vi "PBLV_Interface.vi"() -> ()   [LabVIEW 2012]
uses:
  <vilib>/Utility/error.llb/DialogTypeEnum.ctl
panel:
  in  "board_num":i32
  in  "change board":bool
  in  "# of Instructions":u32=4
  in  "Path to spinapi64.dll":path=path "C:/SpinCore/SpinAPI/dll/spinapi64.dll"
  in  "start/restart":bool
  in  "load":bool
  in  "stop":bool
  in  "clock_freq (MHz)":dbl=100.0
  in  "Instructions":T1(array[cluster])=[{"Instruct Data"=0, "Op Code"=0, "Flags"=[TRUE, FALSE, FALSE, FALSE, FALSE, FALSE, FALSE, FALSE, FALSE, FALSE, FALSE, FALSE, FALSE, FALSE, FALSE, FALSE, FALSE, FALSE, FALSE, FALSE, FALSE, FALSE, FALSE, FALSE], "Comments"="", "Time (s)"=0.1}, {"Instruct Data"=0, "Op Code"=0, "Flags"=[FALSE, FALSE, FALSE, FALSE, FALSE, FALSE, FALSE, FALSE, FALSE, FALSE, FALSE, FALSE, FALSE, FALSE, FALSE, FALSE, FALSE, FALSE, FALSE, FALSE, FALSE, FALSE, FALSE, FALSE], "Comments"="", "Time (s)"=0.1}, {"Instruct Data"=0, "Op Code"=0, "Flags"=[TRUE, FALSE, FALSE, FALSE, FALSE, FALSE, FALSE, FALSE, FALSE, FALSE, FALSE, FALSE, FALSE, FALSE, FALSE, FALSE, FALSE, FALSE, FALSE, FALSE, FALSE, FALSE, FALSE, FALSE], "Comments"="", "Time (s)"=0.1}, {"Instruct Data"=0, "Op Code"=6, "Flags"=[FALSE, FALSE, FALSE, FALSE, FALSE, FALSE, FALSE, FALSE, FALSE, FALSE, FALSE, FALSE, FALSE, FALSE, FALSE, FALSE, FALSE, FALSE, FALSE, FALSE, FALSE, FALSE, FALSE, FALSE], "Comments"="", "Time (s)"=0.1}] {"Time (s)" format="%.3p"; "Op Code" items=["Continue", "Stop", "Loop", "End Loop", "JSR", "RTS", "Branch", "Long Delay", "Wait"]}
  # "LabVIEW PulseBlaster Extension\nPulseBlaster Interface\nSpinCore Technologies, Inc.\nwww.spincore.com"
  # "Caution:    \n            After pressing STOP,\n            all output bits may \nmaintain their final state."
  # "1"
  # "2"
  # "3"
  # "4"
  # "5"
  # "6"
  # "7"
  # "8"
  # "9"
  # "10"
  # "11"
  # "12"
  # "13"
  # "14"
  # "15"
  # "16"
  # "17"
  # "18"
  # "19"
  # "20"
  # "21"
  # "22"
  # "23"
  # "24"
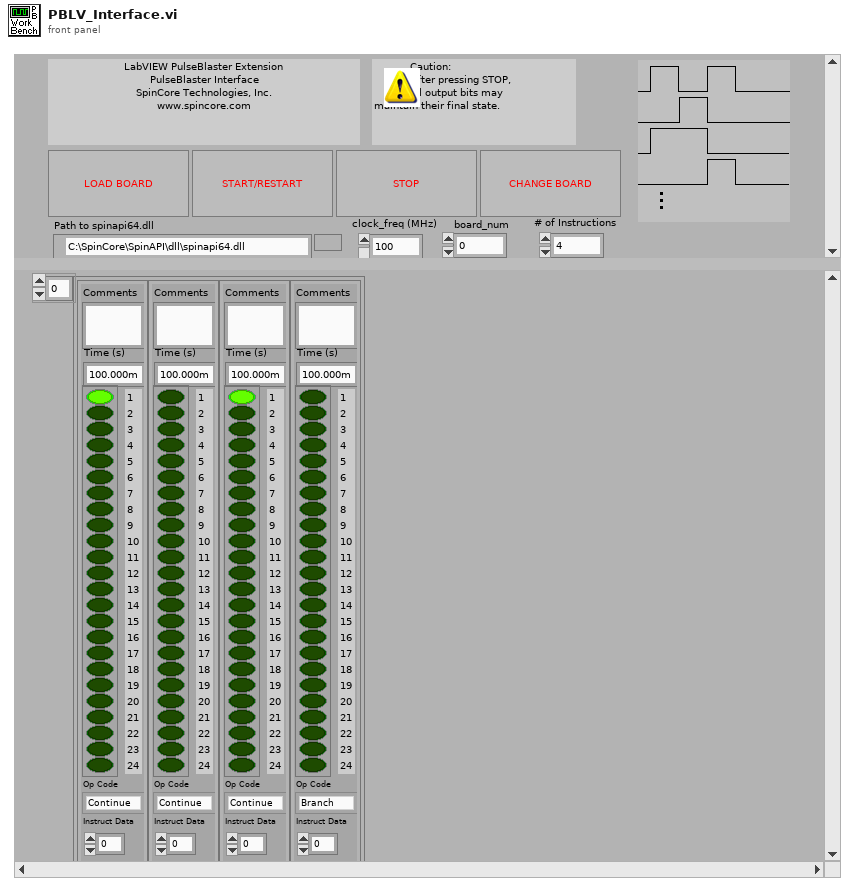
[diagram p1: front panel]
types:
  T1 = cluster{"Instruct Data":i32, "Op Code":i32, "Flags":bool[], "Comments":string, "Time (s)":dbl}[]
  T2 = typedef "DialogTypeEnum.ctl" = enum16{"no dialog", "OK message", "continue or stop message", "auto error handling dialog", "OK message + warnings", "continue/stop + warnings"}
  T3 = enum16{"Pulse Program", "Frequency Registers", "TX Phase Registers", "RX Phase Registers"}
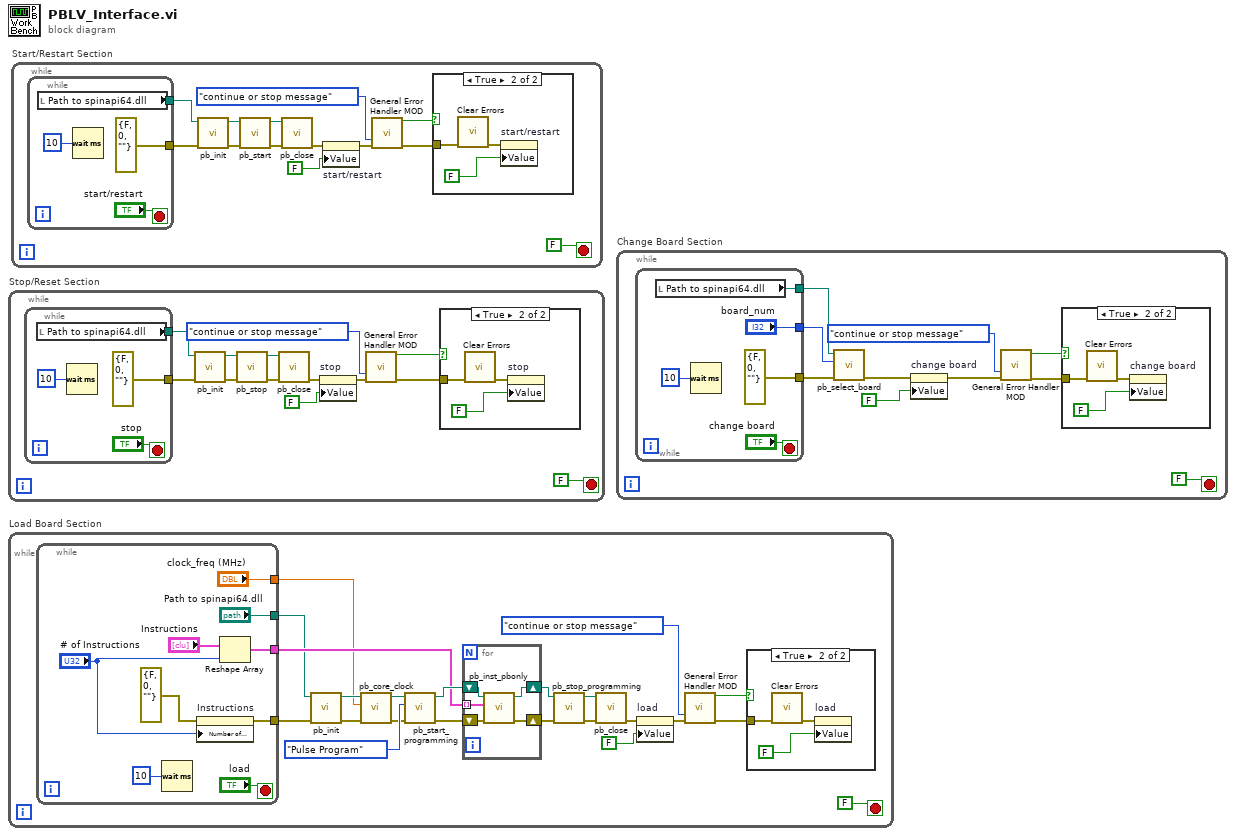
[diagram p0: block diagram]
diagram:
  n1 = while "Stop/Reset Section" {
    stop <- FALSE stop-if-true
    n2 = while {
      tunnel: [errorcluster {"status"=FALSE, "code"=0, "source"=""} ("error in (no error)")] -> w10
      tunnel: [w17] -> w1
      stop <- "stop" stop-if-true
      n3 = local read "Path to spinapi64.dll"() -> (w17:path)
      n4 = Wait (ms)(milliseconds to wait=u32 10) -> ()  [unwired: 1 out]
    }
    n5 = call "pb_init.vi"("error in (no error)"=w10, "path in"=w1) -> ("error out"=w9:errorcluster, "path out"=w12:path)  [unwired: 1 in, 7 out]
    n6 = call "pb_stop.vi"("error in (no error)"=w9, "path in"=w12) -> ("error out"=w8:errorcluster, "path out"=w13:path)  [unwired: 8 out]
    n7 = call "pb_close.vi"("error in (no error)"=w8, "path in"=w13) -> ("error out"=w7:errorcluster)  [unwired: 9 out]
    n8 = property on="stop" class="Bool (strict)"(error in=w7, "Value"=FALSE ("stop")) -> (error out=w6:errorcluster)  [unwired: 1 in, 1 out]
    n9 = call "General Error Handler MOD.vi"("type of dialog (OK msg:1)"=DialogTypeEnum."continue or stop message", "error in (no error)"=w6) -> ("STOP?"=w3:bool, "error out"=w2:errorcluster)  [unwired: 12 out]
    n10 = case shown="True" w3 {
      tunnel: w2 -> [_ w16]
      frame False {
      }
      frame True {
        n11 = call <vilib>:"Clear Errors.vi"("error in (no error)"=w16) -> ("error out"=w14:errorcluster)  [unwired: 6 out]
        n12 = property on="stop" class="Bool (strict)"(error in=w14, "Value"=FALSE ("Waiting for Data Acquisition")) -> ()  [unwired: 1 in, 2 out]
      }
    }
  }
  n13 = while "Load Board Section" {
    stop <- FALSE stop-if-true
    n14 = while {
      tunnel: [w54] -> w37
      tunnel: [w55] -> w39
      tunnel: ["Path to spinapi64.dll"] -> w22
      tunnel: ["clock_freq (MHz)"] -> w21
      stop <- "load" stop-if-true
      n15 = Wait (ms)(milliseconds to wait=u32 10) -> ()  [unwired: 1 out]
      n16 = property on="Instructions" class="Arr (strict)"(error in=errorcluster {"status"=FALSE, "code"=0, "source"=""} ("error in (no error)"), "Number of Columns"="# of Instructions") -> (error out=w54:errorcluster)  [unwired: 1 in, 1 out]
      n17 = Reshape Array("Instructions", "# of Instructions") -> (w55:T1)
    }
    n18 = call "pb_init.vi"("error in (no error)"=w37, "path in"=w22) -> ("error out"=w24:errorcluster, "path out"=w26:path)  [unwired: 2 in, 6 out]
    n19 = call "pb_core_clock.vi"("error in (no error)"=w24, "clock_freq (MHz)"=w21, "path in"=w26) -> ("error out"=w23:errorcluster, "path out"=w25:path)  [unwired: 7 in]
    n20 = call "pb_start_programming.vi"("error in (no error)"=w23, "Device"=T3."Pulse Program", "path in"=w25) -> ("error out"=w35:errorcluster, "path out"=w42:path)  [unwired: 1 in, 6 out]
    n21 = for {
      tunnel: w39 -> [w47] mode=indexing
      shift-right: [w49] -> w38
      shift-left: w42 -> [w50]
      shift-right: [w46] -> w34
      shift-left: w35 -> [w48]
      n22 = call "pb_inst_pbonly.vi"("error in (no error)"=w48, "PB Instruction"=w47, "path in"=w50) -> ("error out"=w46:errorcluster, "path out"=w49:path)  [unwired: 2 in, 5 out]
    }
    n23 = call "pb_stop_programming.vi"("error in (no error)"=w34, "path in"=w38) -> ("error out"=w33:errorcluster, "path out"=w41:path)  [unwired: 1 in, 7 out]
    n24 = call "pb_close.vi"("error in (no error)"=w33, "path in"=w41) -> ("error out"=w31:errorcluster)  [unwired: 9 out]
    n25 = property on="load" class="Bool (strict)"(error in=w31, "Value"=FALSE ("load")) -> (error out=w30:errorcluster)  [unwired: 1 in, 1 out]
    n26 = call "General Error Handler MOD.vi"("type of dialog (OK msg:1)"=DialogTypeEnum."continue or stop message", "error in (no error)"=w30) -> ("STOP?"=w27:bool, "error out"=w28:errorcluster)  [unwired: 12 out]
    n27 = case shown="True" w27 {
      tunnel: w28 -> [_ w45]
      frame False {
      }
      frame True {
        n28 = call <vilib>:"Clear Errors.vi"("error in (no error)"=w45) -> ("error out"=w43:errorcluster)  [unwired: 6 out]
        n29 = property on="load" class="Bool (strict)"(error in=w43, "Value"=FALSE ("Waiting for Data Acquisition")) -> ()  [unwired: 1 in, 2 out]
      }
    }
  }
  n30 = while "Start/Restart Section" {
    stop <- FALSE stop-if-true
    n31 = while {
      tunnel: [errorcluster {"status"=FALSE, "code"=0, "source"=""} ("error in (no error)")] -> w69
      tunnel: [w76] -> w60
      stop <- "start/restart" stop-if-true
      n32 = local read "Path to spinapi64.dll"() -> (w76:path)
      n33 = Wait (ms)(milliseconds to wait=u32 10) -> ()  [unwired: 1 out]
    }
    n34 = call "pb_init.vi"("error in (no error)"=w69, "path in"=w60) -> ("error out"=w68:errorcluster, "path out"=w71:path)  [unwired: 1 in, 7 out]
    n35 = call "pb_start.vi"("error in (no error)"=w68, "path in"=w71) -> ("error out"=w67:errorcluster, "path out"=w72:path)  [unwired: 1 in, 7 out]
    n36 = call "pb_close.vi"("error in (no error)"=w67, "path in"=w72) -> ("error out"=w66:errorcluster)  [unwired: 9 out]
    n37 = property on="start/restart" class="Bool (strict)"(error in=w66, "Value"=FALSE ("start/restart")) -> (error out=w65:errorcluster)  [unwired: 1 in, 1 out]
    n38 = call "General Error Handler MOD.vi"("type of dialog (OK msg:1)"=DialogTypeEnum."continue or stop message", "error in (no error)"=w65) -> ("STOP?"=w62:bool, "error out"=w61:errorcluster)  [unwired: 12 out]
    n39 = case shown="True" w62 {
      tunnel: w61 -> [_ w75]
      frame False {
      }
      frame True {
        n40 = call <vilib>:"Clear Errors.vi"("error in (no error)"=w75) -> ("error out"=w73:errorcluster)  [unwired: 6 out]
        n41 = property on="start/restart" class="Bool (strict)"(error in=w73, "Value"=FALSE ("Waiting for Data Acquisition")) -> ()  [unwired: 1 in, 2 out]
      }
    }
  }
  n42 = while "Change Board Section" {
    stop <- FALSE stop-if-true
    n43 = while {
      tunnel: [errorcluster {"status"=FALSE, "code"=0, "source"=""} ("error in (no error)")] -> w89
      tunnel: ["board_num"] -> w88
      tunnel: [w93] -> w80
      stop <- "change board" stop-if-true
      n44 = local read "Path to spinapi64.dll"() -> (w93:path)
      n45 = Wait (ms)(milliseconds to wait=u32 10) -> ()  [unwired: 1 out]
    }
    n46 = call "pb_select_board.vi"("error in (no error)"=w89, "board_num"=w88, "path in"=w80) -> ("error out"=w86:errorcluster)  [unwired: 8 out]
    n47 = property on="change board" class="Bool (strict)"(error in=w86, "Value"=FALSE ("change board")) -> (error out=w85:errorcluster)  [unwired: 1 in, 1 out]
    n48 = call "General Error Handler MOD.vi"("type of dialog (OK msg:1)"=DialogTypeEnum."continue or stop message", "error in (no error)"=w85) -> ("STOP?"=w82:bool, "error out"=w81:errorcluster)  [unwired: 12 out]
    n49 = case shown="True" w82 {
      tunnel: w81 -> [_ w92]
      frame False {
      }
      frame True {
        n50 = call <vilib>:"Clear Errors.vi"("error in (no error)"=w92) -> ("error out"=w90:errorcluster)  [unwired: 6 out]
        n51 = property on="change board" class="Bool (strict)"(error in=w90, "Value"=FALSE ("Waiting for Data Acquisition")) -> ()  [unwired: 1 in, 2 out]
      }
    }
  }
